vi "GetPosition.vi"(5 "error in":errorcluster, 8 "VISA resource name in":refnum<visa-resource-name>) -> (0 "error out":errorcluster, 1 "Position XYZ":dbl[](array[numeric]), 2 "Number of Bytes":u32, 3 "VISA resource name out":refnum<visa-resource-name>)   [LabVIEW 2016]
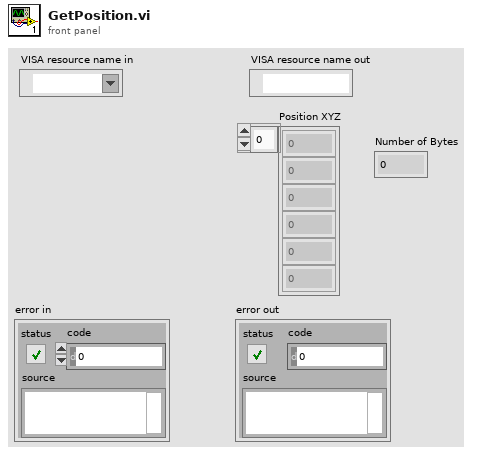
[diagram p1: front panel]
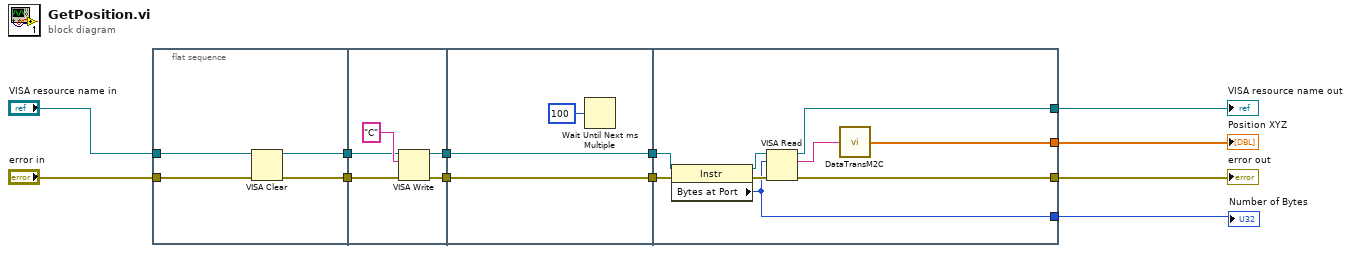
[diagram p0: block diagram]
diagram:
  n1 = flat-sequence {
    tunnel: "error in" -> [w15]
    tunnel: "VISA resource name in" -> [w16]
    tunnel: [w14] -> w3
    tunnel: [w13] -> w2
    tunnel: [w20] -> w7
    tunnel: [w19] -> w5
    tunnel: w3 -> [w18]
    tunnel: w2 -> [w17]
    tunnel: w7 -> [w24]
    tunnel: [w24] -> w6
    tunnel: w5 -> [w23]
    tunnel: [w23] -> w4
    tunnel: w6 -> [w32]
    tunnel: [w31] -> w9
    tunnel: w4 -> [w30]
    tunnel: [w25] -> w8
    tunnel: [w28] -> w10
    tunnel: [w27] -> w1
    frame #0 {
      n2 = VISA Clear(VISA resource name=w16, error in (no error)=w15) -> (VISA resource name out=w14:refnum<visa-resource-name>, error out=w13:errorcluster)
    }
    frame #1 {
      n3 = VISA Write(VISA resource name=w18, write buffer="C", error in (no error)=w17) -> (VISA resource name out=w20:refnum<visa-resource-name>, error out=w19:errorcluster)  [unwired: 1 out]
    }
    frame #2 {
      n4 = Wait Until Next ms Multiple(millisecond multiple=u32 100) -> ()  [unwired: 1 out]
    }
    frame #3 {
      n5 = property class="Instr"(reference=w32, error in=w30) -> (reference out=w33:refnum<visa-resource-name>, error out=w29:errorcluster, "Bytes at Port"=w27:u32)
      n6 = VISA Read(VISA resource name=w33, byte count=w27, error in (no error)=w29) -> (VISA resource name out=w31:refnum<visa-resource-name>, read buffer=w26:string, error out=w25:errorcluster)  [unwired: 1 out]
      n7 = call "DataTransM2C.vi"("MotorData"=w26) -> ("Computer Data"=w28:dbl[])
    }
  }
  "Position XYZ" <- w10
  "VISA resource name out" <- w9
  "error out" <- w8
  "Number of Bytes" <- w1
